vi "Think.vi"(6 "Target":i32, 7 "Target Locations":i32[][](array[numeric]), 8 "Override Engaged":bool, 9 "Current Heading":i32, 10 "Y Position":i32, 11 "X Position":i32) -> (2 "Executable Primitive":string, 3 "Desired Heading":i32, 4 "Desired Y":i32, 5 "Desired X":i32)   [LabVIEW 2012]
uses:
  <vilib>/imath/engines/lvmath/Plug In/_Char/NIMS_CH_character datatype.ctl
  <vilib>/imath/engines/lvmath2/RunTimeEngine/ErrorHandling/NIMS_Finalize Error.vi
  <vilib>/imath/engines/lvmath2/RunTimeEngine/Managers/WorkSpace/UID Generator.vi
  <vilib>/imath/engines/lvmath2/RunTimeEngine/VariableToken/NIMS_VariableToken_CondDefined.vi
  <instcachedir>/0/NIMS_VariableToken_CondDefined_295AAB8C64C949DA8EA45AB7820AF759.lvgen/NIMS_VariableToken_CondDefined_295AAB8C64C949DA8EA45AB7820AF759_003.vi
  <vilib>/imath/engines/lvmath/Plug In/_Char/NIMS_CH_Character RV to String.vi
  <vilib>/imathl/engines/lvmath/Functions/Error Handling/Create Error.vi
  <vilib>/imath/engines/lvmath2/RunTimeEngine/Managers/SymbolTable/Clear UID.vi
  <vilib>/imath/engines/lvmath2/RunTimeEngine/NodeEndStatement/NIMS_NodeEndStatement_Output.vi
  <instcachedir>/0/NIMS_NodeEndStatement_Output_53EC0D466D134D7ABD903AC30B43404B.lvgen/NIMS_NodeEndStatement_Output_53EC0D466D134D7ABD903AC30B43404B_009.vi
  <vilib>/imath/engines/lvmath2/RunTimeEngine/RunTimeType/NIMS_RunTimeType_From StrictType (excl LVString).vi
  <instcachedir>/0/NIMS_RunTimeType_From StrictType (excl LVString)_AC52D965D0864706932D20A05968E122.lvgen/NIMS_RunTimeType_From StrictType (excl LVString)_AC52D965D0864706932D20A05968E122_001.vi
  <vilib>/imath/engines/lvmath2/RunTimeEngine/LocalVariableDefStatement/MC_LocalVariableDefStatement_Display.vi
  <vilib>/imath/engines/lvmath2/RunTimeEngine/Managers/SymbolTable/NIMS_WorkSpace.lvlib
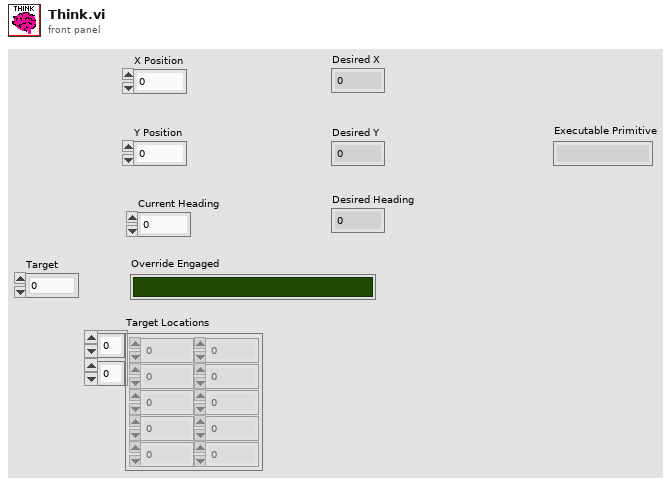
[diagram p1: front panel]
types:
  T1 = typedef "NIMS_CH_character datatype.ctl" = cluster{"Numeric":u8}
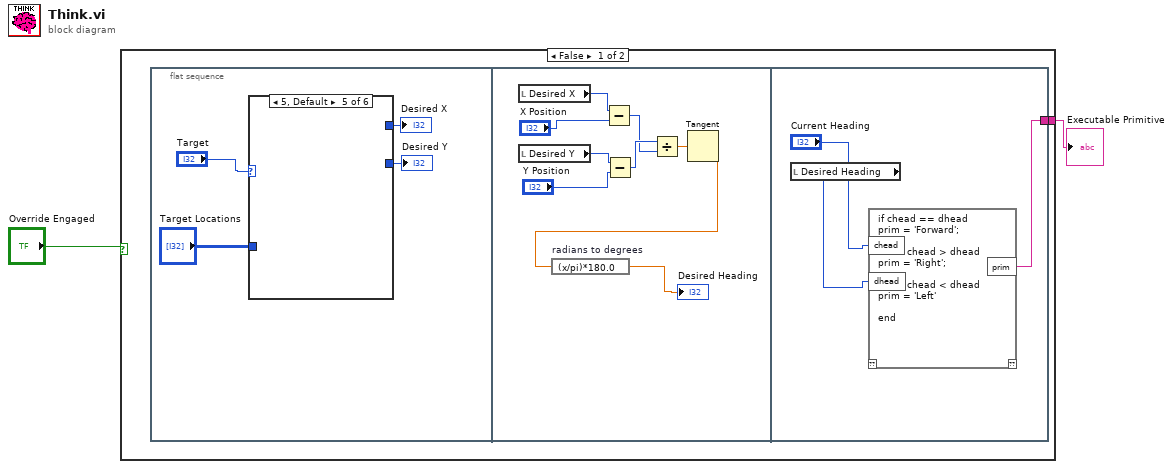
[diagram p0: block diagram]
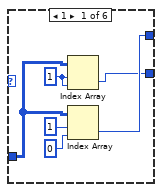
[diagram p2: hidden frame]
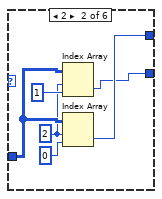
[diagram p3: hidden frame]
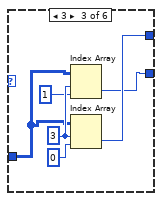
[diagram p4: hidden frame]
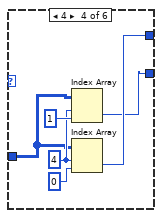
[diagram p5: hidden frame]
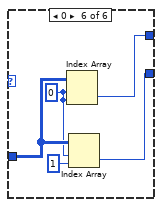
[diagram p6: hidden frame]
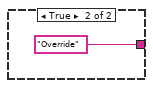
[diagram p7: hidden frame]
diagram:
  n1 = case shown="False" "Override Engaged" {
    tunnel: [w3 "Override"] -> w1
    frame False {
      n2 = flat-sequence {
        tunnel: [w46] -> w3
        frame #0 {
          n3 = case shown="5, Default" "Target" {
            tunnel: "Target Locations" -> [w12 w15 w20 w26 _ w35]
            tunnel: [w11 w17 w22 w28 _ w36] -> w6
            tunnel: [w10 w16 w21 w27 _ w32] -> w5
            frame 1 {
              w8 = 1 ("disabled index (col)")
              n4 = Index Array(array=w12, index (row)=w8, index (col)=w8) -> (element=w10:i32)
              n5 = Index Array(array=w12, index (row)=1, index (col)=0 ("disabled index (col)")) -> (element=w11:i32)
            }
            frame 2 {
              w14 = 2 ("index (row)")
              n6 = Index Array(array=w15, index (row)=w14, index (col)=1 ("disabled index (col)")) -> (element=w16:i32)
              n7 = Index Array(array=w15, index (row)=w14, index (col)=0 ("disabled index (col)")) -> (element=w17:i32)
            }
            frame 3 {
              w25 = 3 ("index (row)")
              n8 = Index Array(array=w20, index (row)=w25, index (col)=1 ("disabled index (col)")) -> (element=w21:i32)
              n9 = Index Array(array=w20, index (row)=w25, index (col)=0 ("disabled index (col)")) -> (element=w22:i32)
            }
            frame 4 {
              w29 = 4 ("index (row)")
              n10 = Index Array(array=w26, index (row)=w29, index (col)=1 ("disabled index (col)")) -> (element=w27:i32)
              n11 = Index Array(array=w26, index (row)=w29, index (col)=0 ("disabled index (col)")) -> (element=w28:i32)
            }
            frame 5, Default {
            }
            frame 0 {
              w34 = 0 ("index (row)")
              n12 = Index Array(array=w35, index (row)=w34, index (col)=w34) -> (element=w36:i32)
              n13 = Index Array(array=w35, index (row)=w34, index (col)=1 ("disabled index (col)")) -> (element=w32:i32)
            }
          }
          "Desired X" <- w6
          "Desired Y" <- w5
        }
        frame #1 {
          n14 = local read "Desired X"() -> (w45:i32)
          n15 = local read "Desired Y"() -> (w43:i32)
          n16 = Subtract(x=w45, y="X Position") -> (x-y=w40:i32)
          n17 = Subtract(x=w43, y="Y Position") -> (x-y=w41:i32)
          n18 = Divide(x=w41, y=w40) -> (x/y=w39:dbl)
          n19 = Tangent(1:w39) -> (0:w38:dbl)
          n20 = expression code="(x/pi)*180.0" "radians to degrees"(w38) -> (→"Desired Heading":dbl)
        }
        frame #2 {
          n21 = local read "Desired Heading"() -> (w47:i32)
          n22 = mathscript code="if chead == dhead\nprim = 'Forward';\n\nelseif chead > dhead\nprim = 'Right';\n\nelseif chead < dhead\nprim = 'Left'\n\nend"("chead"="Current Heading", "dhead"=w47) -> ("prim"=w46:string)  [unwired: 1 in, 1 out]
        }
      }
    }
    frame True {
    }
  }
  "Executable Primitive" <- w1
